vi "Read_binary_data.vi"() -> (0 "Analogue Frequency Hz":dbl format="%.2f", 1 "PWA Binary":i16[][](array[numeric]), 3 "PWA Frequency Hz":dbl format="%.2f", 5 "EOF?":bool, 6 "Block Header":string)   [LabVIEW 2011]
uses:
  Globals/Meas_global.vi
  Globals/LDA_meas_global_1.vi
  Globals/LDA_meas_global_2.vi
panel:
  out "string":string
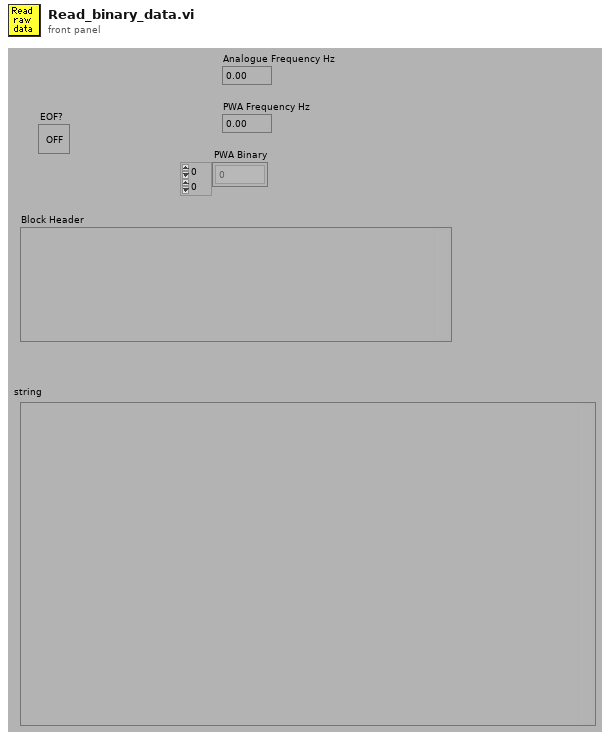
[diagram p1: front panel]
types:
  T1 = enum16{"read/write", "read-only", "write-only", "write-only (truncate)"}
  T2 = typedef "Ch_and_Spans.ctl" = cluster{"high limit (10V)":sgl, "low limit (-10V)":sgl, "Ch No":i16, "Var name":string, "Use Latest Calib":bool}
  T3 = typedef "LDA_Setup.ctl" = cluster{"dimensions":enum16{"1D", "2D"}, "Analogue Freq Multiplier":dbl}
  T4 = typedef "BSA_Type.ctl" = enum16{"57N11", "BSA F60"}
  T5 = typedef "PWA_Data.ctl" = enum16{"No PWA Data", "One Ch PWA"}
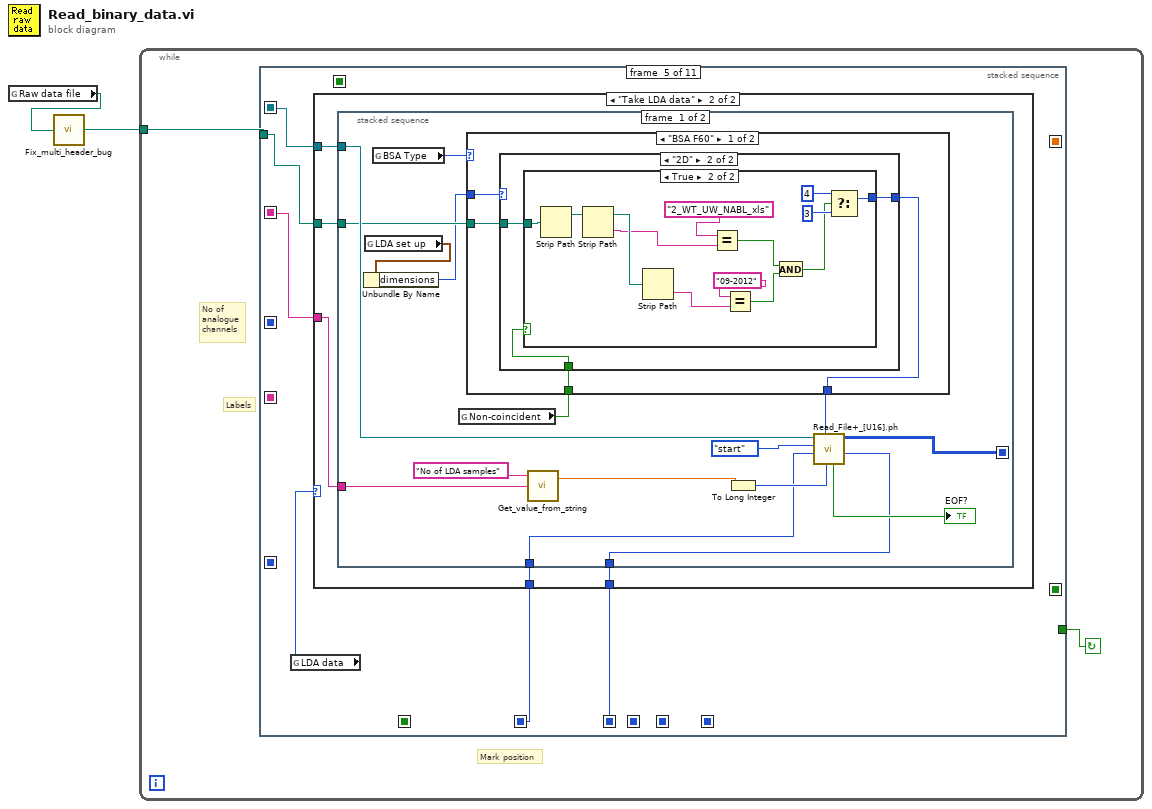
[diagram p0: block diagram]
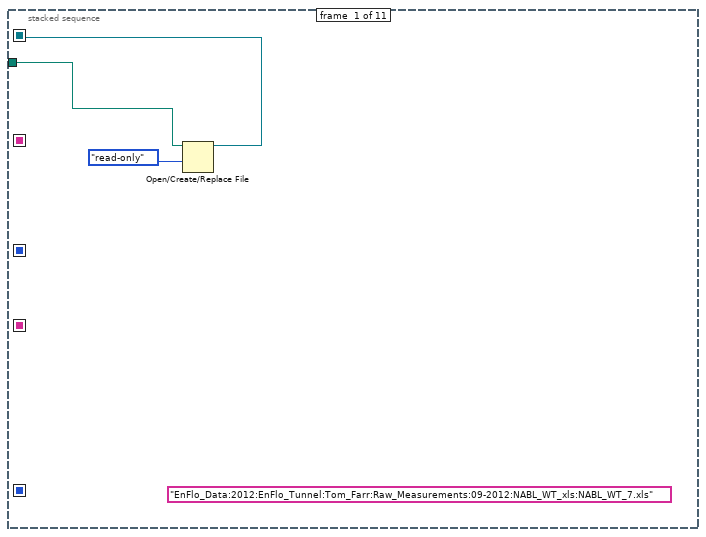
[diagram p2: hidden frame]
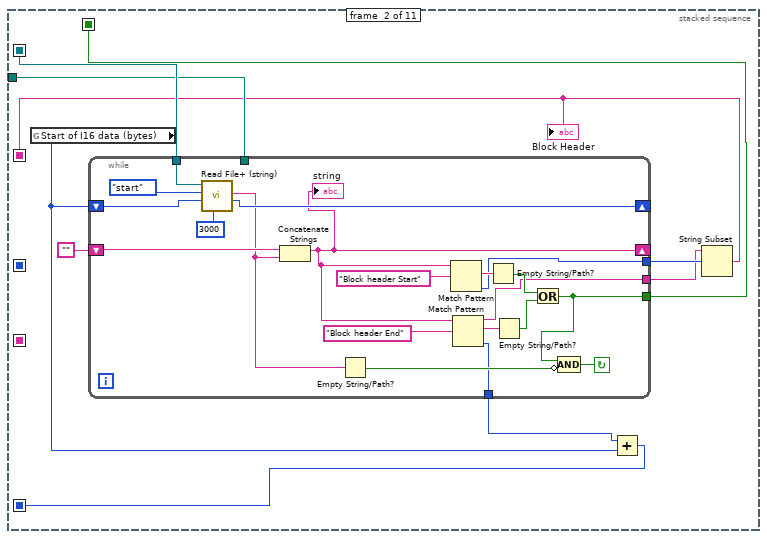
[diagram p3: hidden frame]
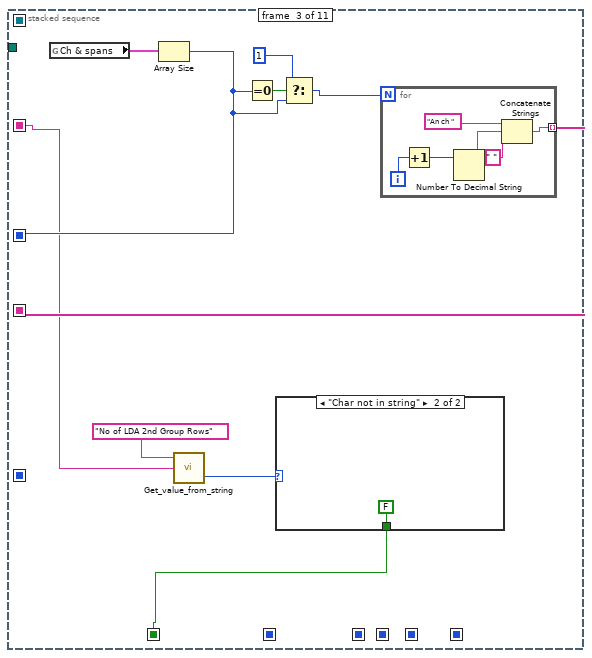
[diagram p4: hidden frame]
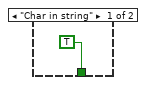
[diagram p5: hidden frame]
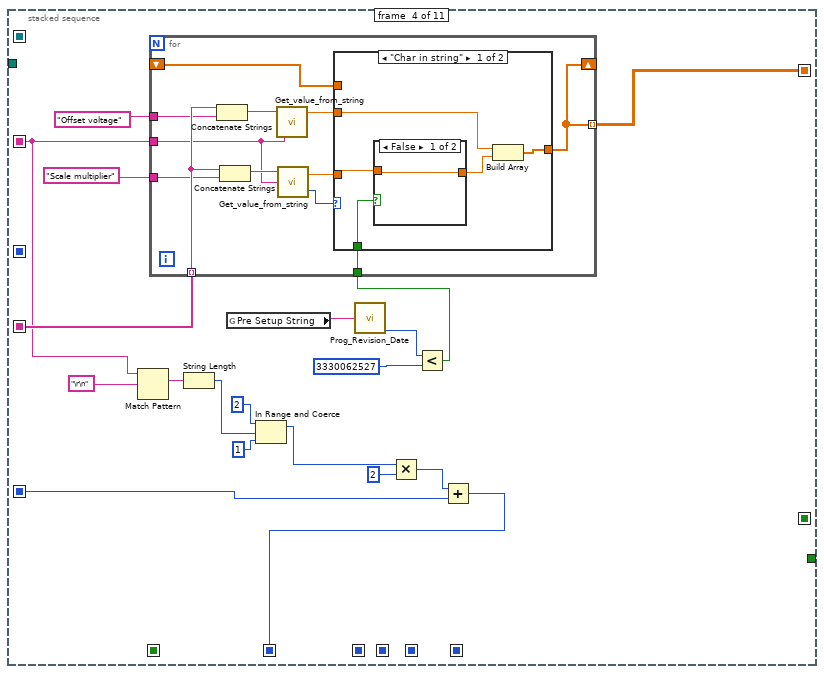
[diagram p6: hidden frame]
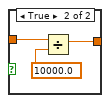
[diagram p7: hidden frame]
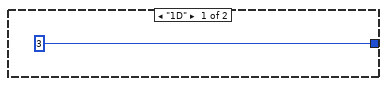
[diagram p10: hidden frame]
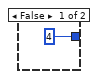
[diagram p11: hidden frame]
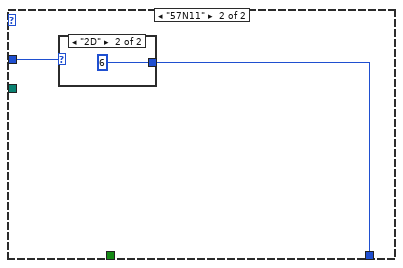
[diagram p12: hidden frame]
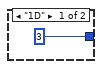
[diagram p13: hidden frame]
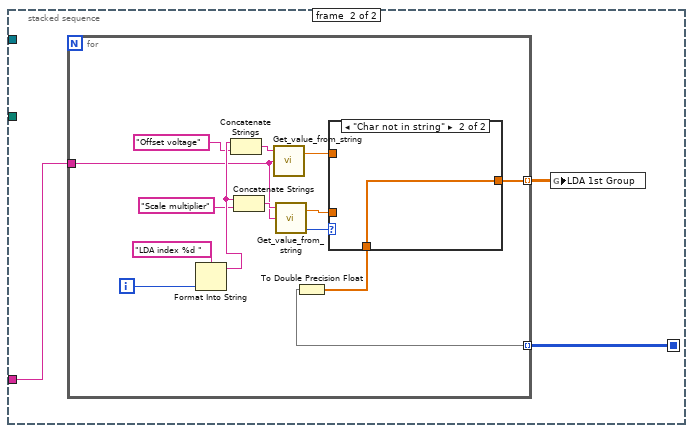
[diagram p14: hidden frame]
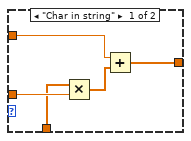
[diagram p15: hidden frame]
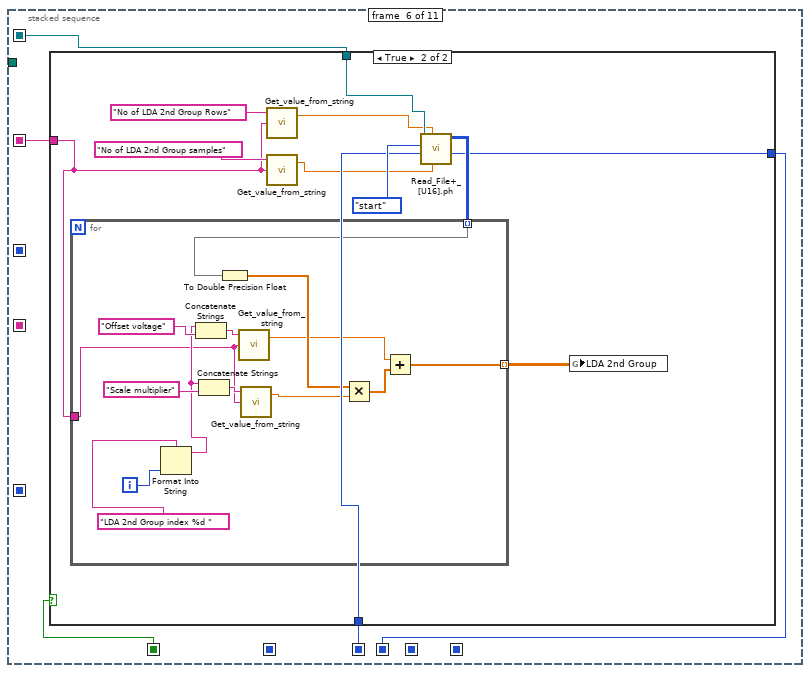
[diagram p16: hidden frame]
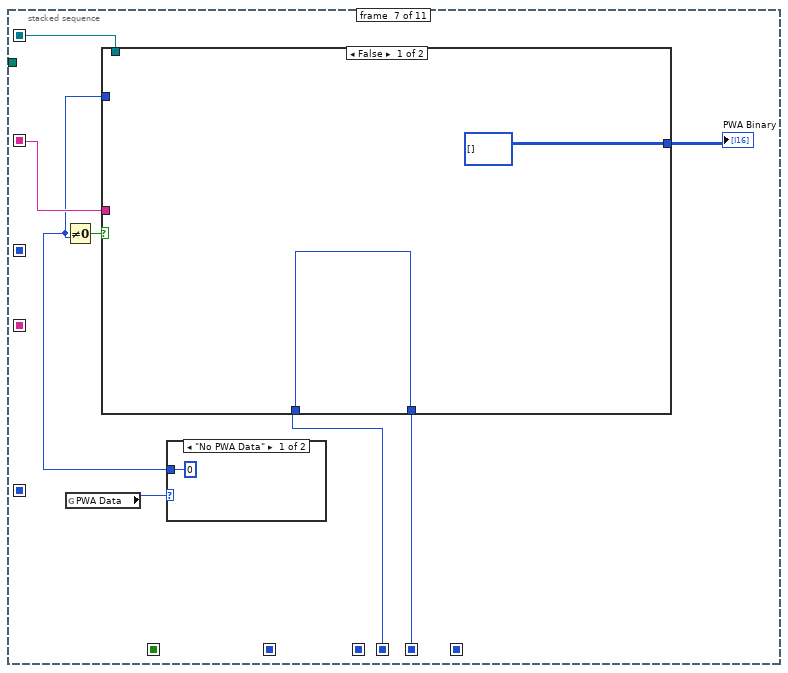
[diagram p18: hidden frame]
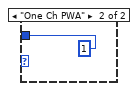
[diagram p19: hidden frame]
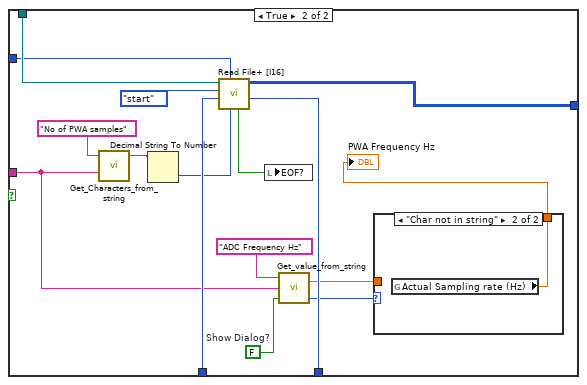
[diagram p20: hidden frame]
diagram:
  n1 = global read "Meas_global.vi" "Raw data file"() -> (w2:path)
  n2 = call "Fix_multi_header_bug.vi"("Raw data File to Read"=w2) -> ("Raw data File to Read Out"=w1:path)
  n3 = while {
    tunnel: w1 -> [w4]
    stop <- w3 continue-if-true
    # "Mark position"
    # "Labels"
    # "No of\nanalogue\nchannels"
    n4 = stacked-sequence {
      seq-local: [w6 _ _ _ _ _ _ _ _ _ _] -> [_ w17 _ _ w99 w176 w210 w242 _ w292 w311]
      seq-local: [_ w8 _ _ _ _ _ _ _ _ _] -> [_ _ w40 w62 w98 w177 w212 w243 w276 _ _]
      seq-local: [_ _ w44 _ _ _ _ _ _ _ _] -> [_ _ _ _ _ _ _ w240 _ _ _]
      seq-local: [_ _ w46 _ _ _ _ _ _ _ _] -> [_ _ _ w74 _ _ _ _ _ _ _]
      seq-local: [_ _ _ w71 _ _ _ _ _ _ _] -> [_ _ _ _ w101 _ _ _ _ _ _]
      seq-local: [_ _ _ _ w100 _ _ _ _ _ _] -> [_ _ _ _ _ w175 _ _ _ _ _]
      seq-local: [_ _ _ _ _ _ w211 _ _ _ _] -> [_ _ _ _ _ _ _ w239 _ _ _]
      seq-local: [_ w13 _ _ _ _ _ _ _ _ _] -> [_ _ _ _ _ _ _ _ _ _ w312]
      seq-local: [_ w12 _ _ _ _ _ _ _ _ _] -> [_ _ _ w72 _ _ _ _ _ _ _]
      seq-local: [_ _ _ _ _ _ _ _ w274 _ _] -> [_ _ _ _ _ _ _ _ _ w290 _]
      seq-local: [_ _ _ _ _ _ _ w238 _ _ _] -> [_ _ _ _ _ _ _ _ w273 w287 _]
      seq-local: [_ _ w38 _ _ _ _ _ _ _ _] -> [_ _ _ _ _ w178 _ _ _ _ _]
      seq-local: [_ _ _ _ _ w174 _ _ _ _ _] -> [_ _ _ _ _ _ w205 _ _ _ _]
      seq-local: [_ _ _ w56 _ _ _ _ _ _ _] -> [_ _ _ _ _ _ _ w235 _ _ _]
      tunnel: w4 -> [w5 w16 _ _ w97 _ _ _ _ _ w313]
      tunnel: [_ _ _ _ _ _ _ _ _ w288 _] -> w3
      frame #0 {
        (unwired) "EnFlo_Data:2012:EnFlo_Tunnel:Tom_Farr:Raw_Measurements:09-2012:NABL_WT_xls:NABL_WT_7.xls"
        n5 = Open/Create/Replace File(file path (use dialog)=w5, access (0:read/write)=T1."read-only" ("open mode (0)")) -> (refnum out=w6:refnum<file>)  [unwired: 1 in, 5 out]
      }
      frame #1 {
        n6 = global read "Meas_global.vi" "Start of I16 data (bytes)"() -> (w14:i32)
        n7 = while {
          tunnel: [w22] -> w11
          tunnel: [w23] -> w13
          shift-left: "" -> [w26]
          shift-right: [w19] -> _
          tunnel: w16 -> [_]
          tunnel: w17 -> [w35]
          shift-left: w14 -> [w29]
          shift-right: [w34] -> _
          tunnel: [w21] -> w9
          tunnel: [w18] -> w10
          stop <- w30 continue-if-true
          n8 = call <vilib>:"Read File+ (string).vi"("count"=3000, "pos offset (bytes:0)"=w29, "pos mode (rel. to current:2)"=enum16{"start", "end", "current"}."start", "refnum"=w35) -> ("mark after read (bytes)"=w34:i32, "string"=w20:string)  [unwired: 1 in, 5 out]
          n9 = Concatenate Strings(w26, w20) -> (w19:string)
          "string" <- w19
          n10 = Empty String/Path?(string/path=w20) -> (empty?=w31:bool)
          n11 = Match Pattern(string=w19, regular expression="Block header Start") -> (match substring=w28:string, offset past match=w18:i32)  [unwired: 3 out]
          n12 = Match Pattern(string=w19, regular expression="Block header End") -> (before substring=w21:string, match substring=w36:string, offset past match=w22:i32)  [unwired: 2 out]
          n13 = Empty String/Path?(string/path=w28) -> (empty?=w25:bool)
          n14 = Empty String/Path?(string/path=w36) -> (empty?=w24:bool)
          n15 = Or(x=w25, y=w24) -> (x .or. y?=w23:bool)
          n16 = Compound Arithmetic op=AND(w23, invert w31) -> (w30:bool)
        }
        n17 = Add(x=w11, y=w14) -> (x+y=w12:i32)
        n18 = String Subset(string=w9, offset (0)=w10) -> (substring=w8:string)  [unwired: 1 out]
        "Block Header" <- w8
      }
      frame #2 {
        n19 = global read "Meas_global.vi" "Ch & spans"() -> (w47:T2[])
        n20 = Array Size(array=w47) -> (size(s)=w44:i32)
        n21 = call "Get_value_from_string.vi"("Input string"=w40, "Variable name"="No of LDA 2nd Group Rows") -> ("Status"=w39:enum16{"Char in string", "Char not in string"})  [unwired: 1 in, 1 out]
        n22 = Equal To 0?(x=w44) -> (x = 0?=w45:bool)
        n23 = case shown="\"Char not in string\"" w39 {
          tunnel: [TRUE FALSE] -> w38
          frame "Char in string" {
          }
          frame "Char not in string" {
          }
        }
        n24 = Select(t=1, s=w45, f=w44) -> (s? t:f=w42:i32)
        n25 = for {
          N: w42 -> [_]
          tunnel: [w51] -> w46 mode=indexing
          i -> [w53]
          n26 = Increment(x=w53) -> (x+1=w52:i32)
          n27 = Number To Decimal String(number=w52) -> (decimal integer string=w55:string)  [unwired: 1 out]
          n28 = Concatenate Strings("An ch ", w55, " ") -> (w51:string)
        }
      }
      frame #3 {
        n29 = Match Pattern(string=w62, regular expression="\r\n") -> (match substring=w61:string)  [unwired: 4 out]
        n30 = String Length(string=w61) -> (length=w60:i32)
        n31 = global read "Meas_global.vi" "Pre Setup String"() -> (w66:string)
        n32 = In Range and Coerce(upper limit=2, x=w60, lower limit=1) -> (coerced(x)=w59:i32)  [unwired: 1 out]
        n33 = call "Prog_Revision_Date.vi"("Input string"=w66) -> ("Revision time (s)"=w67:u32)  [unwired: 4 out]
        n34 = Multiply(x=w59, y=2) -> (x*y=w68:i32)
        n35 = Less?(x=w67, y=u32 3330062527 ("unsigned 32bit integer")) -> (x < y?=w64:bool)
        n36 = for {
          tunnel: w74 -> [w86] mode=indexing
          tunnel: "Scale multiplier" -> [w85]
          tunnel: "Offset voltage" -> [w84]
          tunnel: w62 -> [w81]
          tunnel: [w77] -> w56 mode=indexing
          shift-right: [w77] -> _
          shift-left: _ -> [w78]
          tunnel: w64 -> [w75]
          n37 = Concatenate Strings(w86, w84) -> (w83:string)
          n38 = Concatenate Strings(w86, w85) -> (w82:string)
          n39 = call "Get_value_from_string.vi"("Input string"=w81, "Variable name"=w83) -> ("Value"=w79:dbl)  [unwired: 1 in, 1 out]
          n40 = call "Get_value_from_string.vi"("Input string"=w81, "Variable name"=w82) -> ("Status"=w76:enum16{"Char in string", "Char not in string"}, "Value"=w80:dbl)  [unwired: 1 in]
          n41 = case shown="\"Char in string\"" w76 {
            tunnel: w80 -> [w91 _]
            tunnel: w79 -> [w90 _]
            tunnel: [w88 w96] -> w77
            tunnel: w78 -> [_ w96]
            tunnel: w75 -> [w87 _]
            frame "Char in string" {
              n42 = case shown="False" w87 {
                tunnel: w91 -> [w92 w95]
                tunnel: [w92 w93] -> w89
                frame False {
                }
                frame True {
                  n43 = Divide(x=w95, y=10000.0) -> (x/y=w93:dbl)
                }
              }
              n44 = Build Array(w90, w89) -> (w88:dbl[])
            }
            frame "Char not in string" {
            }
          }
        }
        n45 = Add(x=w68, y=w72) -> (x+y=w71:i32)
      }
      frame #4 {
        n46 = global read "Meas_global.vi" "LDA data"() -> (w102:enum16{"No LDA data", "Take LDA data"})
        n47 = case shown="\"Take LDA data\"" w102 {
          tunnel: w98 -> [_ w106]
          tunnel: w101 -> [w103 w107]
          tunnel: [w103 w105] -> w100
          tunnel: w99 -> [_ w108]
          tunnel: w97 -> [_ w104]
          frame "No LDA data" {
          }
          frame "Take LDA data" {
            n48 = stacked-sequence {
              seq-local: [w111 _] -> [_ w152]
              tunnel: w108 -> [w124 _]
              tunnel: w107 -> [w116 _]
              tunnel: w106 -> [w115 w153]
              tunnel: [w113 _] -> w105
              tunnel: w104 -> [w112 _]
              frame #0 {
                n49 = global read "Meas_global.vi" "LDA set up"() -> (w110:T3)
                n50 = Unbundle By Name(w110) -> ("dimensions"=w109:enum16{"1D", "2D"})
                n51 = global read "LDA_meas_global_1.vi" "BSA Type"() -> (w118:T4)
                n52 = global read "LDA_meas_global_1.vi" "Non-coincident"() -> (w114:bool)
                n53 = case shown="\"BSA F60\"" w118 {
                  tunnel: w109 -> [w128 w148]
                  tunnel: [w126 w147] -> w117
                  tunnel: w114 -> [w127 _]
                  tunnel: w112 -> [w125 _]
                  frame "BSA F60" {
                    n54 = case shown="\"2D\"" w128 {
                      tunnel: [3 w132] -> w126
                      tunnel: w127 -> [_ w131]
                      tunnel: w125 -> [_ w130]
                      frame "1D" {
                      }
                      frame "2D" {
                        n55 = case shown="True" w131 {
                          tunnel: [4 w144] -> w132
                          tunnel: w130 -> [_ w143]
                          frame False {
                          }
                          frame True {
                            n56 = Strip Path(path=w143) -> (stripped path=w141:path)  [unwired: 1 out]
                            n57 = Strip Path(path=w141) -> (stripped path=w142:path, name=w138:string)
                            n58 = Strip Path(path=w142) -> (name=w137:string)  [unwired: 1 out]
                            n59 = Equal?(x="2_WT_UW_NABL_xls", y=w138) -> (x = y?=w135:bool)
                            n60 = Equal?(x="09-2012", y=w137) -> (x = y?=w136:bool)
                            n61 = And(x=w135, y=w136) -> (x .and. y?=w134:bool)
                            n62 = Select(t=4, s=w134, f=3) -> (s? t:f=w144:i32)
                          }
                        }
                      }
                    }
                  }
                  frame "57N11" {
                    n63 = case shown="\"2D\"" w148 {
                      tunnel: [3 6] -> w147
                      frame "1D" {
                      }
                      frame "2D" {
                      }
                    }
                  }
                }
                n64 = call "Get_value_from_string.vi"("Input string"=w115, "Variable name"="No of LDA samples") -> ("Value"=w122:dbl)  [unwired: 1 in, 1 out]
                n65 = To Long Integer(number=w122) -> (32bit integer=w120:i32)
                n66 = call "Read_File+_[U16].ph.vi"("2D number of columns/1D count"=w120, "2D number of rows"=w117, "pos offset (bytes:0)"=w116, "pos mode (rel. to current:2)"=enum16{"start", "end", "current"}."start", "refnum"=w124) -> ("mark after read (bytes)"=w113:i32, "2D data"=w111:u16[][], "EOF?"=→"EOF?":bool)  [unwired: 1 in, 3 out]
              }
              frame #1 {
                n67 = for {
                  tunnel: w153 -> [w159]
                  tunnel: w152 -> [w157] mode=indexing
                  tunnel: [w155] -> w151 mode=indexing
                  i -> [w158]
                  n68 = Format Into String(format string="LDA index %d ", w158) -> (resulting string=w164:string)  [unwired: 2 in, 1 out]
                  n69 = Concatenate Strings(w164, "Offset voltage") -> (w161:string)
                  n70 = Concatenate Strings(w164, "Scale multiplier") -> (w160:string)
                  n71 = call "Get_value_from_string.vi"("Input string"=w159, "Variable name"=w161) -> ("Value"=w165:dbl)  [unwired: 1 in, 1 out]
                  n72 = call "Get_value_from_string.vi"("Input string"=w159, "Variable name"=w160) -> ("Status"=w154:enum16{"Char in string", "Char not in string"}, "Value"=w167:dbl)  [unwired: 1 in]
                  n73 = To Double Precision Float(number=w157) -> (double precision float=w156:dbl[])
                  n74 = case shown="\"Char not in string\"" w154 {
                    tunnel: w167 -> [w172 _]
                    tunnel: w165 -> [w171 _]
                    tunnel: w156 -> [w169 w173]
                    tunnel: [w168 w173] -> w155
                    frame "Char in string" {
                      n75 = Multiply(x=w169, y=w172) -> (x*y=w170:dbl[])
                      n76 = Add(x=w171, y=w170) -> (x+y=w168:dbl[])
                    }
                    frame "Char not in string" {
                    }
                  }
                }
                n77 = global write "LDA_meas_global_2.vi" "LDA 1st Group"(w151) -> ()
              }
            }
          }
        }
      }
      frame #5 {
        n78 = case shown="True" w178 {
          tunnel: w177 -> [_ w185]
          tunnel: w176 -> [_ w187]
          tunnel: w175 -> [w179 w186]
          tunnel: [w179 w183] -> w174
          frame False {
          }
          frame True {
            n79 = call "Get_value_from_string.vi"("Input string"=w185, "Variable name"="No of LDA 2nd Group Rows") -> ("Value"=w182:dbl)  [unwired: 1 in, 1 out]
            n80 = call "Get_value_from_string.vi"("Input string"=w185, "Variable name"="No of LDA 2nd Group samples") -> ("Value"=w181:dbl)  [unwired: 1 in, 1 out]
            n81 = call "Read_File+_[U16].ph.vi"("2D number of columns/1D count"=w181, "2D number of rows"=w182, "pos offset (bytes:0)"=w186, "pos mode (rel. to current:2)"=enum16{"start", "end", "current"}."start", "refnum"=w187) -> ("mark after read (bytes)"=w183:i32, "2D data"=w184:u16[][])  [unwired: 1 in, 4 out]
            n82 = for {
              tunnel: w185 -> [w199]
              tunnel: w184 -> [w192] mode=indexing
              tunnel: [w191] -> w180 mode=indexing
              i -> [w195]
              n83 = Format Into String(format string="LDA 2nd Group index %d ", w195) -> (resulting string=w200:string)  [unwired: 2 in, 1 out]
              n84 = Concatenate Strings(w200, "Offset voltage") -> (w203:string)
              n85 = Concatenate Strings(w200, "Scale multiplier") -> (w204:string)
              n86 = To Double Precision Float(number=w192) -> (double precision float=w198:dbl[])
              n87 = call "Get_value_from_string.vi"("Input string"=w199, "Variable name"=w203) -> ("Value"=w196:dbl)  [unwired: 1 in, 1 out]
              n88 = call "Get_value_from_string.vi"("Input string"=w199, "Variable name"=w204) -> ("Value"=w194:dbl)  [unwired: 1 in, 1 out]
              n89 = Multiply(x=w198, y=w194) -> (x*y=w197:dbl[])
              n90 = Add(x=w196, y=w197) -> (x+y=w191:dbl[])
            }
            n91 = global write "LDA_meas_global_2.vi" "LDA 2nd Group"(w180) -> ()
          }
        }
      }
      frame #6 {
        n92 = global read "Meas_global.vi" "PWA Data"() -> (w208:T5)
        n93 = case shown="\"No PWA Data\"" w208 {
          tunnel: [0 1] -> w207
          frame "No PWA Data" {
          }
          frame "One Ch PWA" {
          }
        }
        n94 = Not Equal To 0?(x=w207) -> (x != 0?=w209:bool)
        n95 = case shown="False" w209 {
          tunnel: w212 -> [_ w220]
          tunnel: w205 -> [w216 w225]
          tunnel: [w216 w227] -> w211
          tunnel: w210 -> [_ w231]
          tunnel: w207 -> [_ w230]
          tunnel: [i16[][] [] ("2D array") w226] -> w206
          frame False {
          }
          frame True {
            w221 = FALSE  # Show Dialog?
            n96 = call "Get_Characters_from_string.vi"("Input string"=w220, "Variable name"="No of PWA samples") -> ("Value"=w224:string)  [unwired: 1 in, 1 out]
            n97 = Decimal String To Number(string=w224) -> (number=w223:i32)  [unwired: 3 out]
            n98 = call <vilib>:"Read File+ [I16].vi"("2D number of columns/1D count"=w223, "2D number of rows"=w230, "pos offset (bytes:0)"=w225, "pos mode (rel. to current:2)"=enum16{"start", "end", "current"}."start", "refnum"=w231) -> ("mark after read (bytes)"=w227:i32, "2D data"=w226:i16[][], "EOF?"=w228:bool)  [unwired: 1 in, 3 out]
            n99 = local write "EOF?"(w228) -> ()
            n100 = call "Get_value_from_string.vi"("Show Dialog?"=w221, "Input string"=w220, "Variable name"="ADC Frequency Hz") -> ("Status"=w219:enum16{"Char in string", "Char not in string"}, "Value"=w218:dbl)
            n101 = case shown="\"Char not in string\"" w219 {
              tunnel: w218 -> [w233 _]
              tunnel: [w233 w234] -> w217
              frame "Char in string" {
              }
              frame "Char not in string" {
                n102 = global read "Meas_global.vi" "Actual Sampling rate (Hz)"() -> (w234:dbl)
              }
            }
            "PWA Frequency Hz" <- w217
          }
        }
        "PWA Binary" <- w206
      }
      frame #7 {
        n103 = Not Equal To 0?(x=w240) -> (x != 0?=w241:bool)
        n104 = case shown="True" w241 {
          tunnel: w243 -> [_ w258]
          tunnel: w239 -> [w254 w263]
          tunnel: [w254 w265] -> w238
          tunnel: w242 -> [_ w269]
          tunnel: w240 -> [_ w268]
          tunnel: [i16[][] [] ("2D array") w264] -> w237
          frame False {
          }
          frame True {
            w259 = FALSE  # Show Dialog?
            n105 = call "Get_Characters_from_string.vi"("Input string"=w258, "Variable name"="No of Analogue samples") -> ("Value"=w262:string)  [unwired: 1 in, 1 out]
            n106 = Decimal String To Number(string=w262) -> (number=w261:i32)  [unwired: 3 out]
            n107 = call <vilib>:"Read File+ [I16].vi"("2D number of columns/1D count"=w261, "2D number of rows"=w268, "pos offset (bytes:0)"=w263, "pos mode (rel. to current:2)"=enum16{"start", "end", "current"}."start", "refnum"=w269) -> ("mark after read (bytes)"=w265:i32, "2D data"=w264:i16[][], "EOF?"=w266:bool)  [unwired: 1 in, 3 out]
            n108 = local write "EOF?"(w266) -> ()
            n109 = call "Get_value_from_string.vi"("Show Dialog?"=w259, "Input string"=w258, "Variable name"="ADC Frequency Hz") -> ("Status"=w257:enum16{"Char in string", "Char not in string"}, "Value"=w256:dbl)
            n110 = case shown="\"Char not in string\"" w257 {
              tunnel: w256 -> [w271 _]
              tunnel: [w271 w272] -> w255
              frame "Char in string" {
              }
              frame "Char not in string" {
                n111 = global read "Meas_global.vi" "Actual Sampling rate (Hz)"() -> (w272:dbl)
              }
            }
            "Analogue Frequency Hz" <- w255
          }
        }
        n112 = for {
          tunnel: [w244] -> w236 mode=indexing
          tunnel: w237 -> [w251] mode=indexing
          tunnel: w235 -> [w247] mode=indexing
          n113 = To Double Precision Float(number=w251) -> (double precision float=w250:dbl[])
          n114 = Index Array(array=w247, index=0) -> (element=w246:dbl)
          n115 = Index Array(array=w247, index=1) -> (element=w245:dbl)
          n116 = Multiply(x=w250, y=w245) -> (x*y=w252:dbl[])
          n117 = Add(x=w246, y=w252) -> (x+y=w244:dbl[])
        }
        n118 = global write "Meas_global.vi" "Analogue volts"(w236) -> ()
      }
      frame #8 {
        n119 = global read "Meas_global.vi" "Blocks to Skip"() -> (w275:i32[])
        n120 = Array Size(array=w275) -> (size(s)=w278:i32)
        n121 = Equal To 0?(x=w278) -> (x = 0?=w277:bool)
        n122 = case shown="False" w277 {
          tunnel: w276 -> [w284 _]
          tunnel: w275 -> [w281 _]
          tunnel: [w279 FALSE] -> w274
          frame False {
            n123 = call "Get_value_from_string.vi"("Input string"=w284, "Variable name"="Block No") -> ("Value"=w283:dbl)  [unwired: 1 in, 1 out]
            n124 = To Long Integer(number=w283) -> (32bit integer=w282:i32)
            n125 = Search 1D Array(1D array=w281, element=w282) -> (index of element=w280:i32)  [unwired: 1 out]
            n126 = Greater Or Equal To 0?(x=w280) -> (x >= 0?=w279:bool)
          }
          frame True {
          }
        }
        n127 = global write "Meas_global.vi" "Start of I16 data (bytes)"(w273) -> ()
      }
      frame #9 {
        n128 = local read "EOF?"() -> (w291:bool)
        n129 = case shown="False" w291 {
          tunnel: w287 -> [w295 _]
          tunnel: w292 -> [w294 _]
          tunnel: [w293 w309] -> w289
          tunnel: w291 -> [_ w309]
          frame False {
            n130 = while {
              tunnel: [w299] -> w293
              tunnel: w294 -> [w306]
              shift-left: w295 -> [w301]
              shift-right: [w302] -> _
              stop <- w297 continue-if-true
              n131 = call <vilib>:"Read File+ (string).vi"("count"=3000, "pos offset (bytes:0)"=w301, "pos mode (rel. to current:2)"=enum16{"start", "end", "current"}."start", "refnum"=w306) -> ("error out"=w300:errorcluster, "mark after read (bytes)"=w302:i32, "string"=w303:string, "EOF?"=w296:bool)  [unwired: 1 in, 3 out]
              n132 = Unbundle By Name(w300) -> ("status"=w298:bool)
              n133 = Match Pattern(string=w303, regular expression="Block header") -> (match substring=w307:string)  [unwired: 4 out]
              n134 = Empty String/Path?(string/path=w307) -> (empty?=w299:bool)
              n135 = Compound Arithmetic op=AND(w299, invert w298, invert w296) -> (w297:bool)
            }
          }
          frame True {
          }
        }
        n136 = local write "EOF?"(w289) -> ()
        n137 = Compound Arithmetic op=AND(w290, invert w289) -> (w288:bool)
      }
      frame #10 {
        n138 = Close File(refnum=w311) -> (error out=w310:errorcluster)  [unwired: 1 in, 1 out]
        n139 = case shown="False" w312 {
          tunnel: w313 -> [w316 _]
          tunnel: w310 -> [w314 _]
          frame False {
            n140 = call "Add_filename_to_err_message.vi"("error in (no error)"=w314, "Path"=w316) -> ("error out"=w317:errorcluster)
            n141 = call "EnFlo_Error_Handler.vi"("error in (no error)"=w317, "Dialog Box (T)"=TRUE) -> ()  [unwired: 1 in, 3 out]
          }
          frame True {
            w321 = FALSE  # Dialog Box
            n142 = Bundle By Name(cluster=errorcluster {"status"=FALSE, "code"=0, "source"=""} ("error in (no error)"), "status"=TRUE ("Bundle Element"), "source"="The block header was not found in the file" ("Bundle Element")) -> (w322:errorcluster)
            n143 = call "EnFlo_Error_Handler.vi"("error in (no error)"=w322, "Error Type"="Raw Data File Error", "Dialog Box (T)"=w321) -> ()  [unwired: 3 out]
          }
        }
      }
    }
  }
